vi "CreateODS.vi"() -> ()   [LabVIEW 2013]
uses:
  <userlib>/_OpenG.lib/lvzip/lvzip.llb/ZLIB Open ZIP Mode__ogtk.ctl
  <userlib>/_OpenG.lib/lvzip/lvzip.llb/ZLIB Open Zip Archive__ogtk.vi
  <userlib>/_OpenG.lib/file/file.llb/Compare Two Paths - Scalar__ogtk.vi
panel:
  in  "Folder Path":path=path "C:/Users/Steve Watts/Desktop/ISO9000/Checklist/ddd - Copy"
  out "error out":errorcluster
  out "Files":path[](array[path])=[path "C:/Users/Steve Watts/Desktop/ISO9000/Checklist/ddd - Copy/content.xml", path "C:/Users/Steve Watts/Desktop/ISO9000/Checklist/ddd - Copy/manifest.rdf", path "C:/Users/Steve Watts/Desktop/ISO9000/Checklist/ddd - Copy/meta.xml", path "C:/Users/Steve Watts/Desktop/ISO9000/Checklist/ddd - Copy/mimetype", path "C:/Users/Steve Watts/Desktop/ISO9000/Checklist/ddd - Copy/settings.xml", path "C:/Users/Steve Watts/Desktop/ISO9000/Checklist/ddd - Copy/styles.xml", path "C:/Users/Steve Watts/Desktop/ISO9000/Checklist/ddd - Copy/Configurations2/accelerator/current.xml", path "C:/Users/Steve Watts/Desktop/ISO9000/Checklist/ddd - Copy/META-INF/manifest.xml", path "C:/Users/Steve Watts/Desktop/ISO9000/Checklist/ddd - Copy/Thumbnails/thumbnail.png"]
  in  "Archive":path=path "C:/Users/Steve Watts/Desktop/ISO9000/Checklist/ddd - Copy"
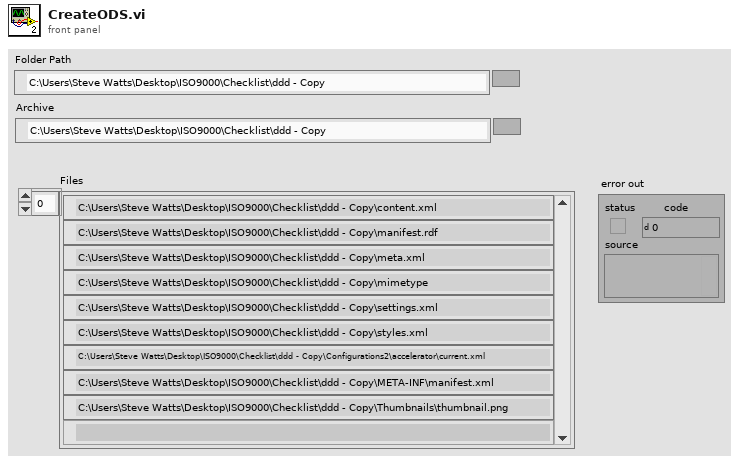
[diagram p1: front panel]
types:
  T1 = typedef "ZLIB Open ZIP Mode__ogtk.ctl" = enum16{"create new", "append to end", "append to archive"}
  T2 = typedef "ZLIB Zip Handle__ogtk.ctl" = refnum<k1>
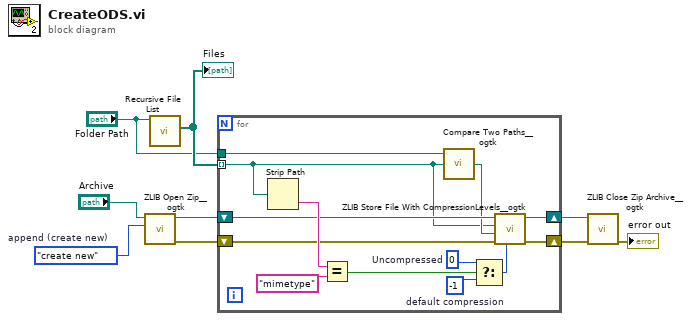
[diagram p0: block diagram]
diagram:
  w9 = ZLIB_Open_ZIP_Mode__ogtk."create new"  # append (create new)
  n1 = call-poly <userlib>:"ZLIB Open Zip__ogtk.vi"("append (create new)"=w9, "archive name"="Archive") -> ("error out"=w6:errorcluster, "zip Refnum"=w7:T2)  [unwired: 3 in, 1 out]
  n2 = call <vilib>:"Recursive File List.vi"("Folder Path"="Folder Path") -> ("All Files in Dir"=w2:path[])  [unwired: 6 in, 4 out]
  "Files" <- w2
  n3 = for {
    shift-right: [w13] -> w5
    shift-left: w7 -> [w16]
    shift-right: [w12] -> w4
    shift-left: w6 -> [w11]
    tunnel: w2 -> [w14] mode=indexing
    tunnel: "Folder Path" -> [w17]
    w18 = -1  # default compression
    w19 = 0  # Uncompressed
    n4 = Strip Path(path=w14) -> (name=w22:string)  [unwired: 1 out]
    n5 = Equal?(x=w22, y="mimetype") -> (x = y?=w20:bool)
    n6 = call-poly <userlib>:"Compare Two Paths__ogtk.vi"("path2"=w14, "path1"=w17) -> ("relative path from 1 to 2"=w15:path)  [unwired: 1 in, 2 out]
    n7 = Select(t=w19, s=w20, f=w18) -> (s? t:f=w10:i32)
    n8 = call "ZLIB Store File With CompressionLevels__ogtk.vi"("-1: use default\ncompression"=w10, "error in (no error)"=w11, "internal name (same as source name)"=w15, "source path"=w14, "zip Refnum"=w16) -> ("error out"=w12:errorcluster, "zip Refnum out"=w13:T2)  [unwired: 5 in]
  }
  n9 = call <userlib>:"ZLIB Close Zip Archive__ogtk.vi"("error in (no error)"=w4, "zip Refnum"=w5) -> ("error out"=→"error out":errorcluster)  [unwired: 4 in, 1 out]
